vi "浊度电极校准.vi"() -> ()   [LabVIEW 2016, in "斯坦道多参数.lvlib"]
uses:
  <vilib>/Utility/miscctls.llb/LVPointTypeDef.ctl
  <vilib>/Utility/miscctls.llb/LVPositionTypeDef.ctl
  <vilib>/Analysis/NI_AALBase.lvlib
panel:
  in  "刷新按钮":bool
  out "第三点信号值":dbl
  out "第二点信号值":dbl
  out "第一点信号值":dbl
  out "温度":dbl format="%#.2f"
  out "通讯状态":string
  out "电极状态标志":u16(ring) items=["OK"=0, "第一点校正通过"=1, "第二点校正通过"=2, "悬浮物两点校准第一点校正通过"=11, "悬浮物两点校准第二点校正通过"=12, "浊度三点校正第一点校正通过"=31, "浊度三点校正第二点校正通过"=32, "浊度三点校正第三点校正通过"=33]
  out "第三点校准值":dbl
  out "标液3":dbl
  out "第二点校准值":dbl
  out "第一点校准值":dbl
  in  "校准停止":bool
  in  "校准启动":bool
  in  "校准模式":u16(ring) items=["两点校准", "单点校准", "三点校准"]
  out "最小值":sgl format="%#.2f"
  out "最大值":sgl format="%#.2f"
  out "波形图表":dbl(graph) caption="历史曲线"
  out "mean":dbl caption="均值" format="%#.2f"
  out "standard deviation":dbl caption="标准差" format="%#.2f"
  out "变异系数":dbl format="%#.6f"
  out "测量值":dbl format="%#.2f"
  out "提示":string
  out "标液2":dbl
  out "标液1":dbl
  out "信号值":dbl format="%#.2f"
  out "偏移值补偿":dbl caption="浊度偏移修正值" format="%#.2f"
  out "电极斜率":dbl format="%#.6f"
  out "电极零点":dbl format="%#.6f"
  # "浊度电极设定"
  # "℃"
  # "NTU"
  # "%"
  # "请选择校准模式:"
  # "NTU"
  # "NTU"
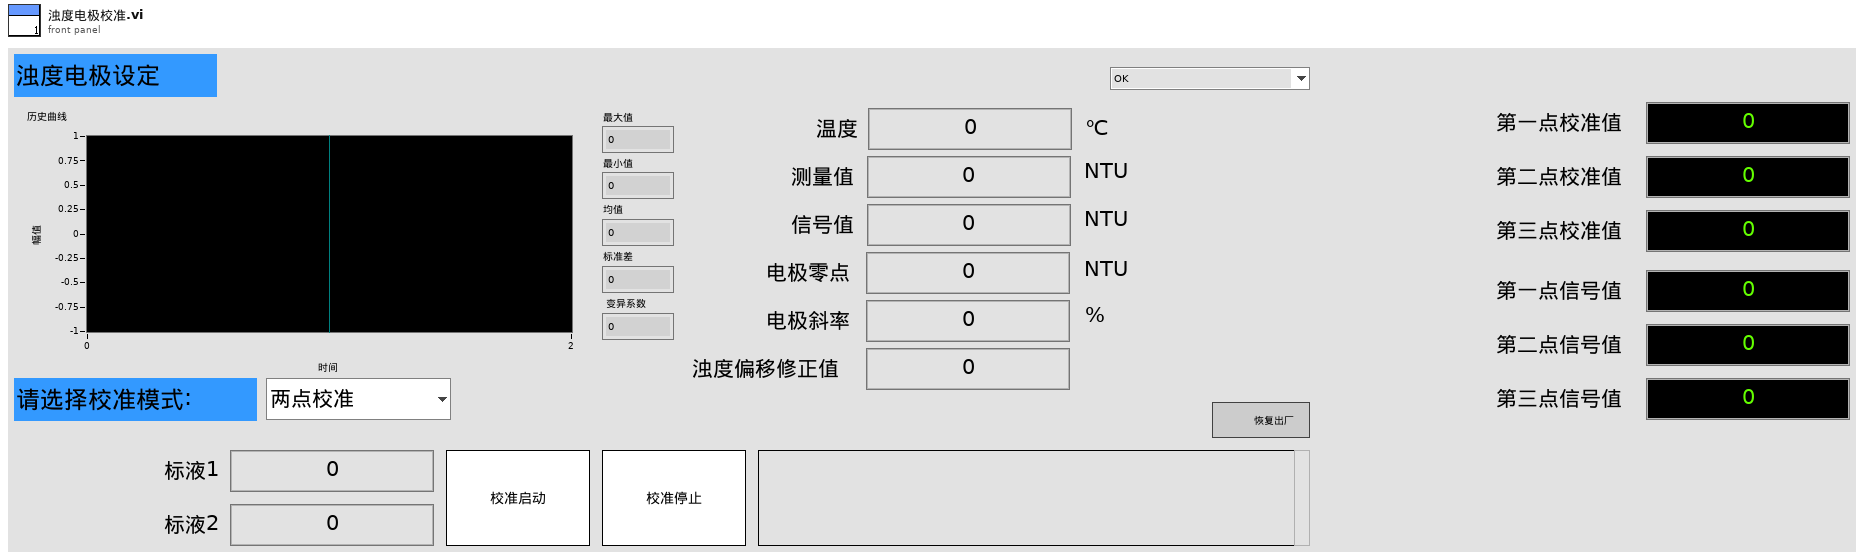
[diagram p1: front panel]
types:
  T1 = typedef "LVPointTypeDef.ctl" = cluster{"Horizontal":i16, "Vertical":i16}
  T2 = cluster{"电极状态标志":u16, "电极型号标志":u16, "浊度测量值":sgl, "温度测量值":sgl, "浊度信号值":sgl, "浊度偏移修正值":sgl, "温度偏移修正值":sgl, "手动温度补偿值":sgl, "浊度电极零点":sgl, "浊度电极斜率":sgl, "第1点标准值记录":sgl, "第1点信号值记录":sgl, "第1点温度值记录":sgl, "第2点标准值记录":sgl, "第2点信号值记录":sgl, "第2点温度值记录":sgl, "命令滤波设定":u16, "温度模式":enum16{"ATC", "MTC"}, "生产批次":u16, "电极序号":u16, "串口地址":u16, "串口波特率":enum16{"9600", "19200", "115200"}, "串口校验位":enum16{"NONE", "ODD", "EVEN"}, "串口停止位":enum16{"1bit", "2bit"}, "第一点标准值":sgl, "第二点标准值":sgl, "第三点标准值":sgl}
  T3 = typedef "LVPositionTypeDef.ctl" = cluster{"Left":i32, "Top":i32}
  T4 = enum8{"Enabled", "Disabled", "Disabled and Grayed Out"}
  T5 = cluster{"测量量程":dbl, "测量精度":dbl, "测量间隔":dbl, "消解温度":dbl, "消解时长":dbl, "空白校准时间":timestamp, "曲线截距":dbl, "曲线斜率":dbl, "测量检出限":dbl, "测量信号值":dbl, "线性相关系数":dbl, "二次多项式系数":dbl, "标样校准时间":timestamp, "单位":enum16{"ug/L", "mg/L"}}
  T6 = cluster{"ph":bool, "DO":bool, "Cond":bool, "Turb":bool, "叶绿素a":bool, "藻密度":bool, "ORP":bool}
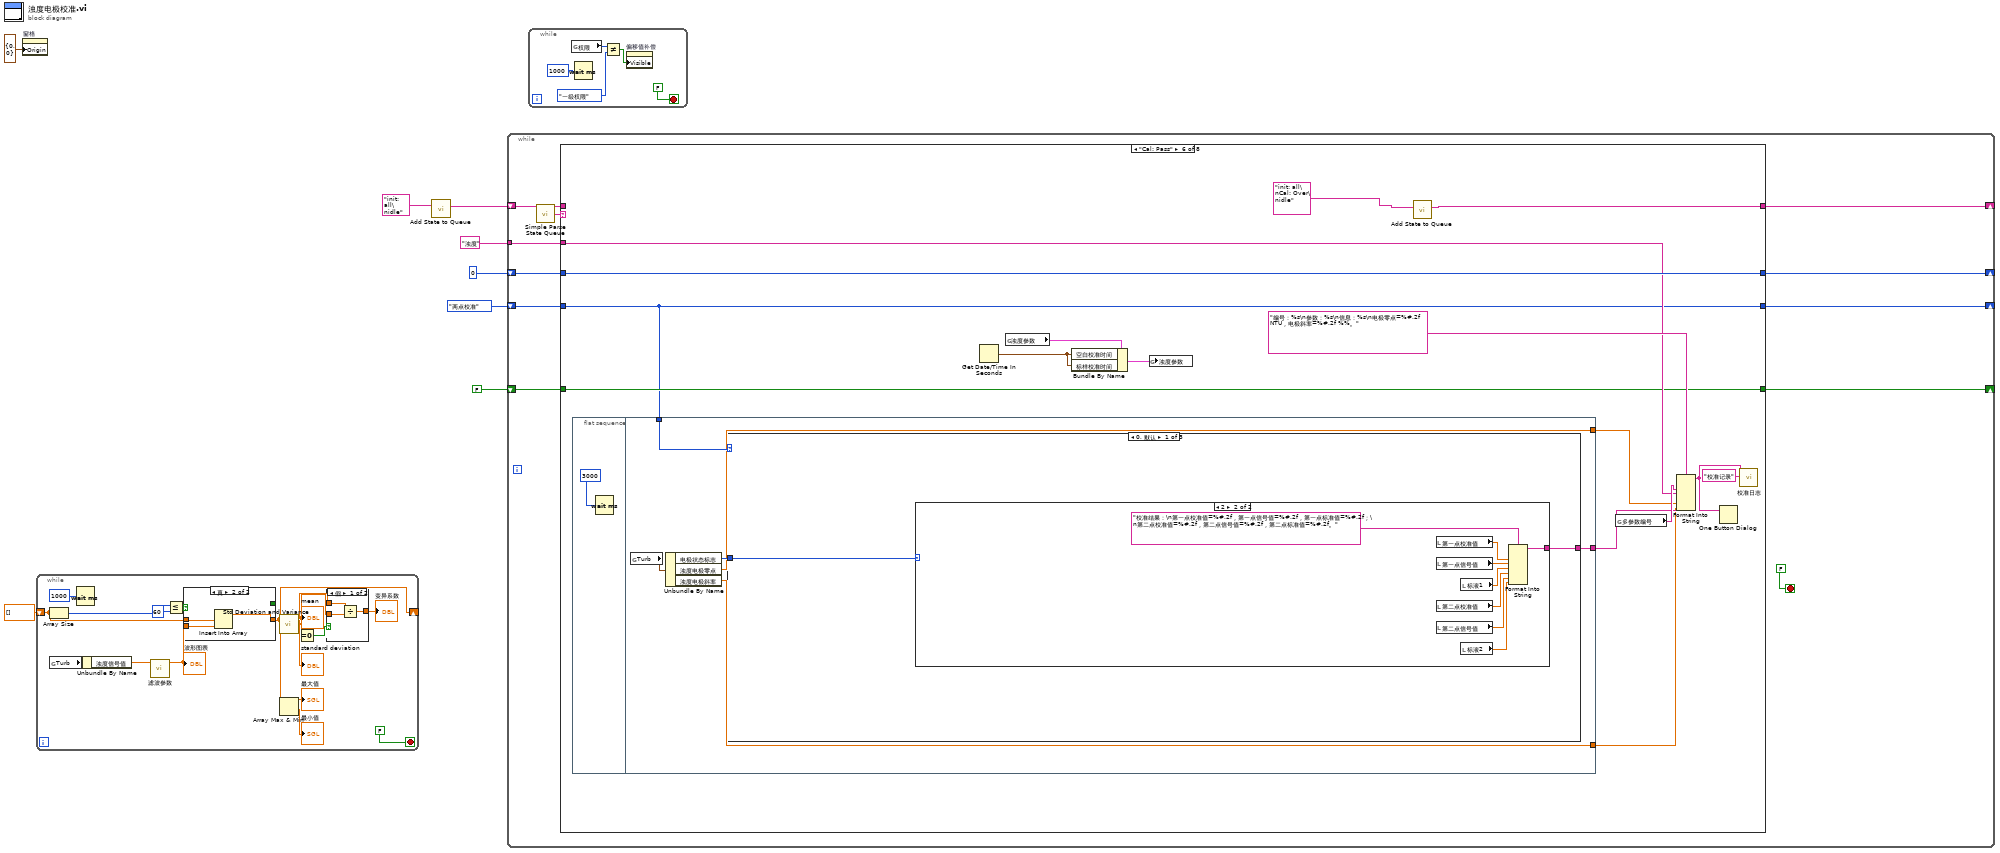
[diagram p0: block diagram]
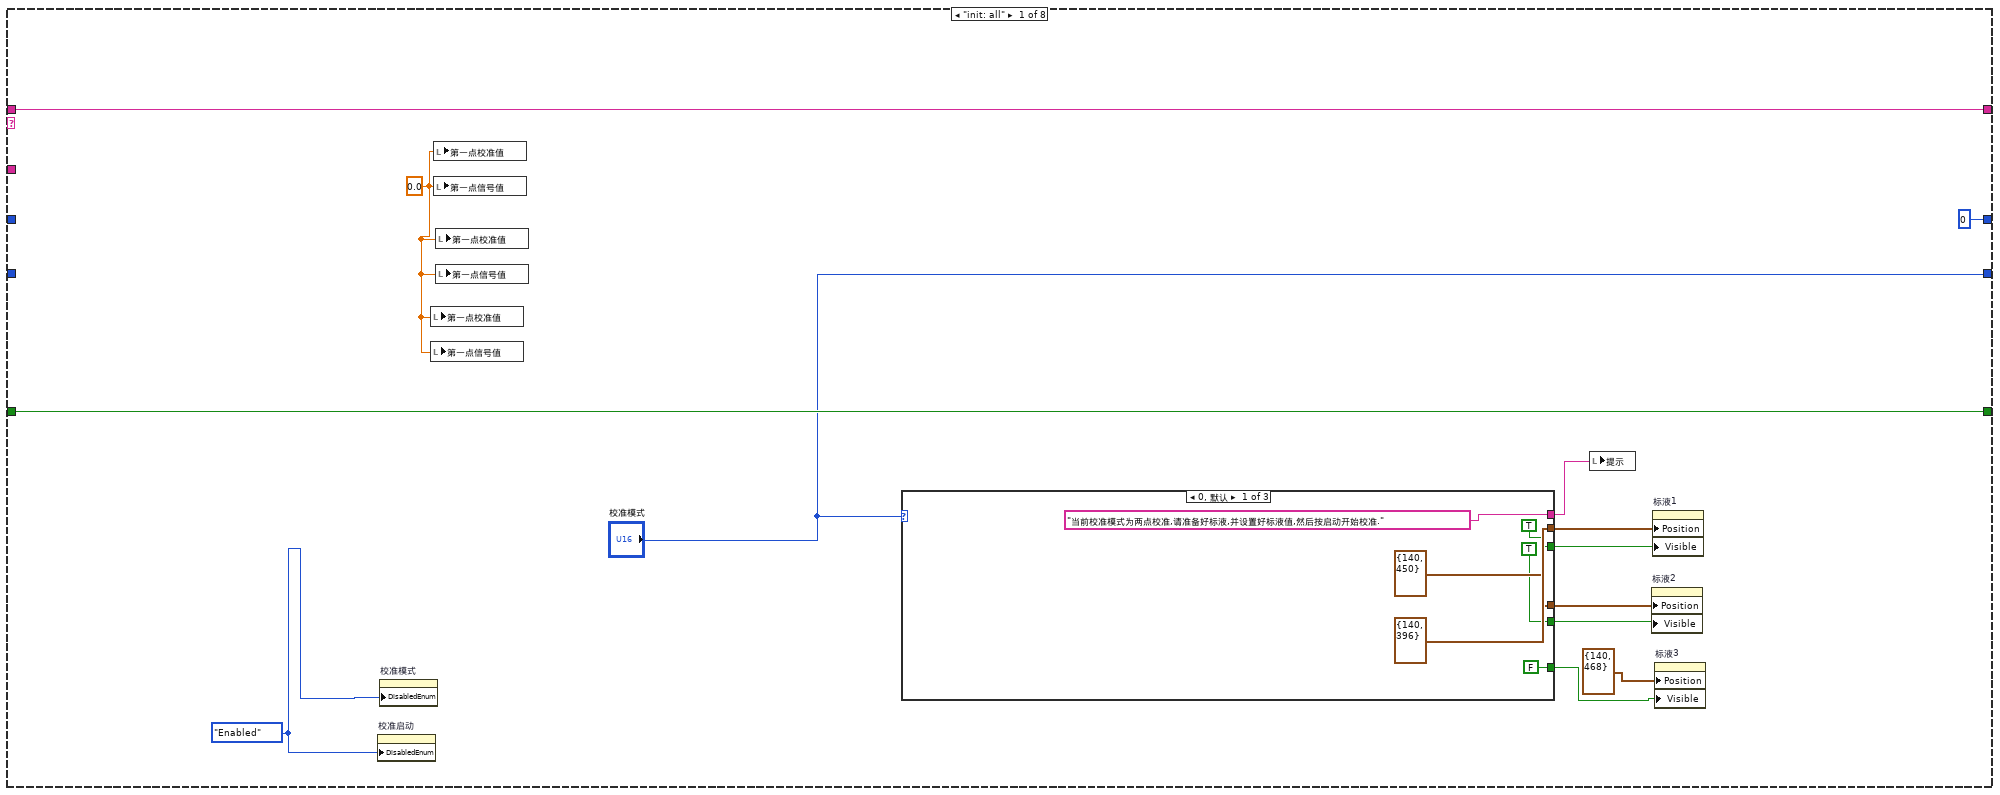
[diagram p2: hidden frame]
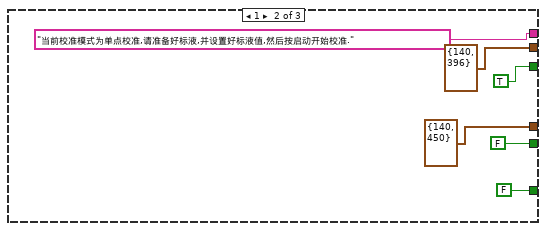
[diagram p3: hidden frame]
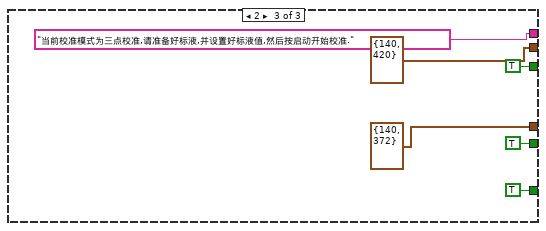
[diagram p4: hidden frame]
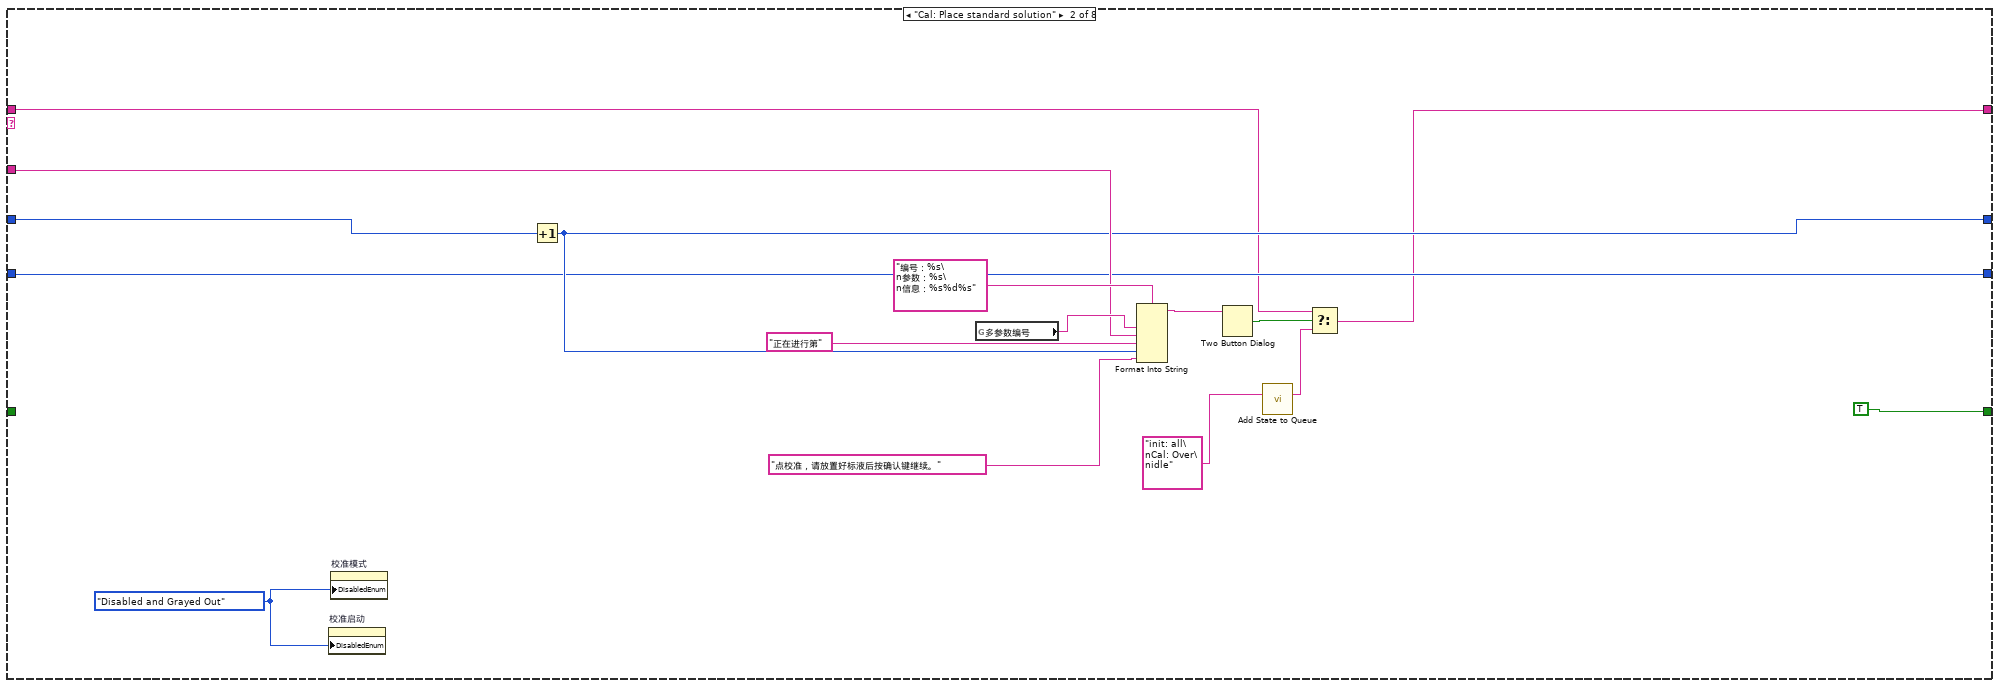
[diagram p5: hidden frame]
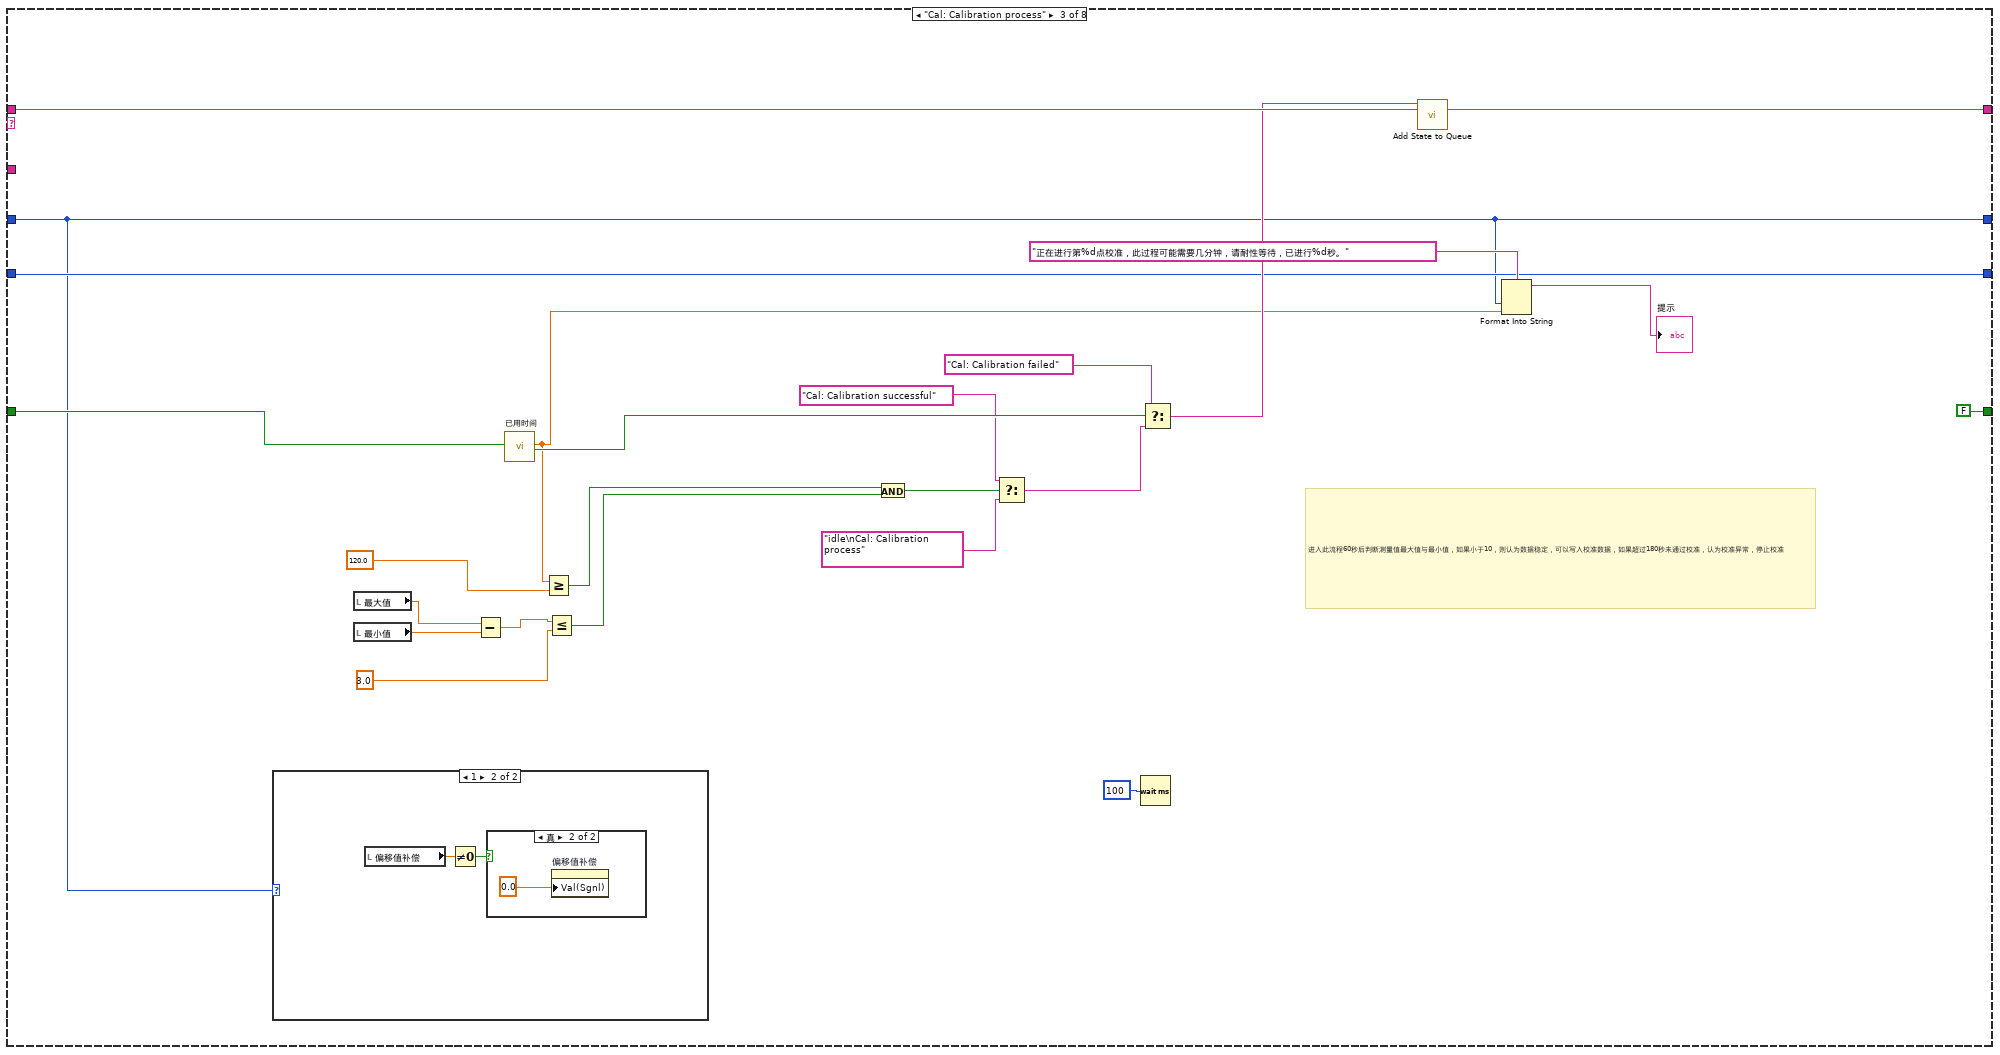
[diagram p6: hidden frame]
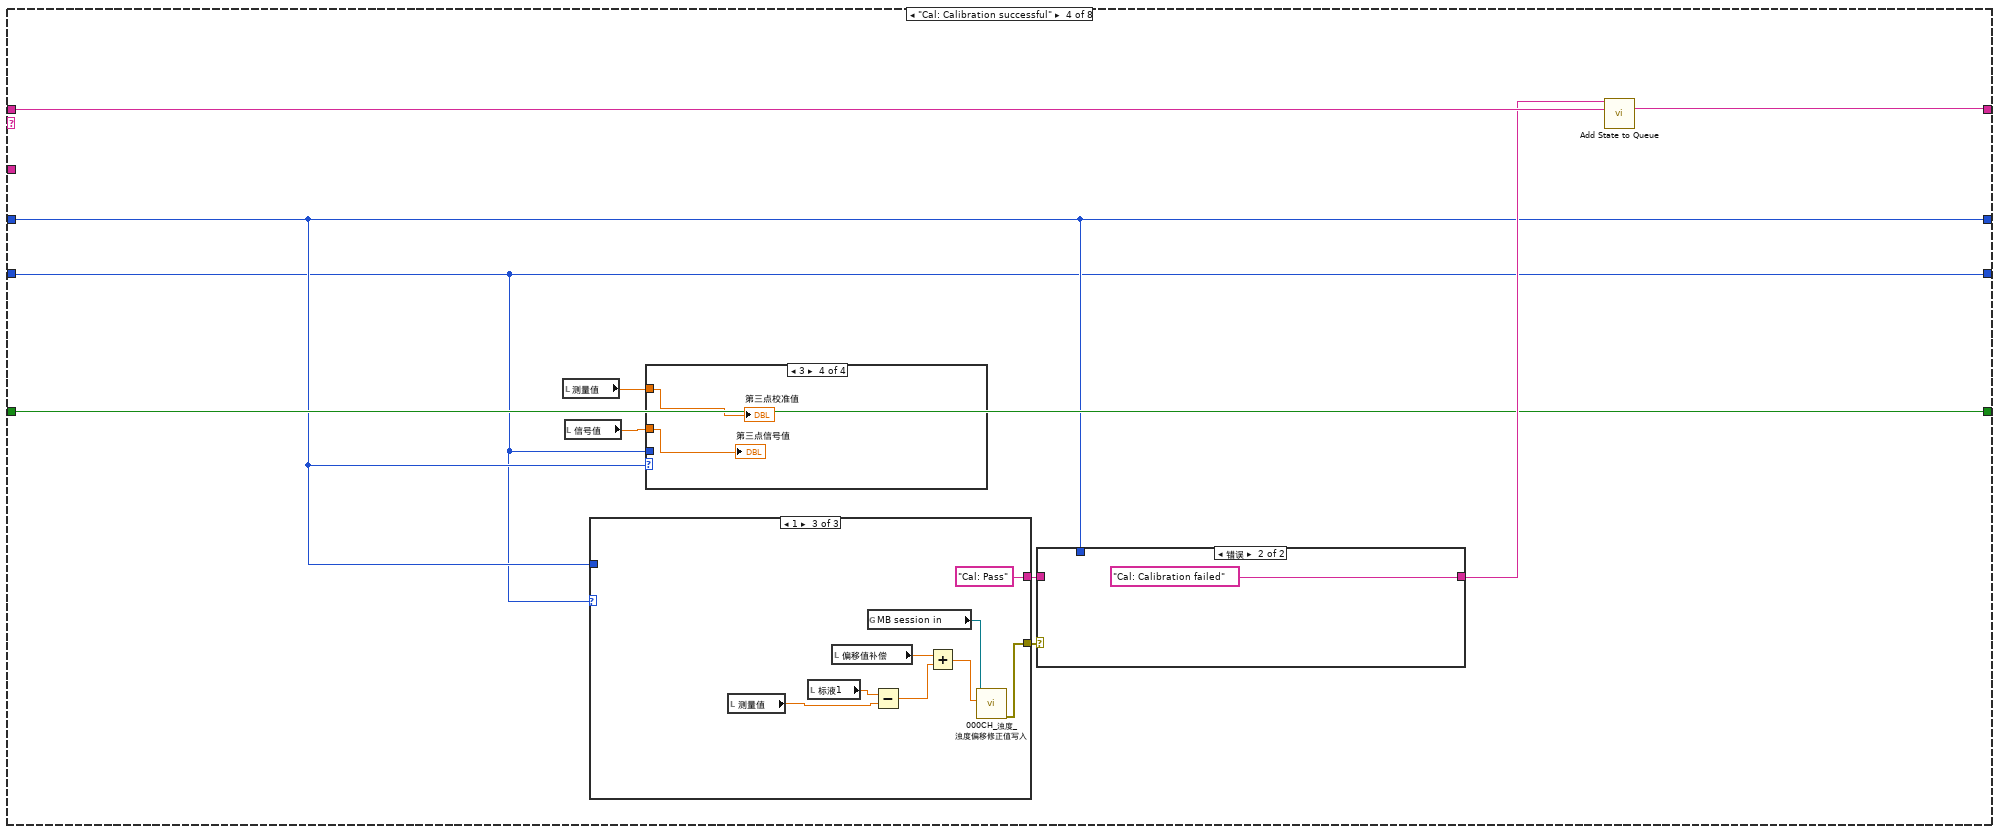
[diagram p9: hidden frame]
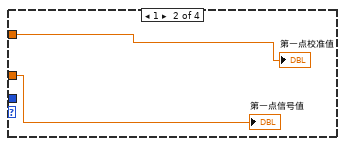
[diagram p11: hidden frame]
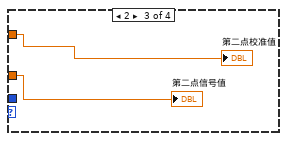
[diagram p12: hidden frame]
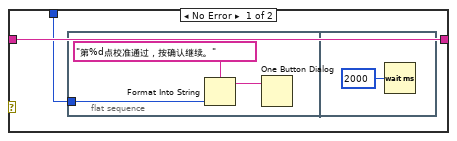
[diagram p13: hidden frame]
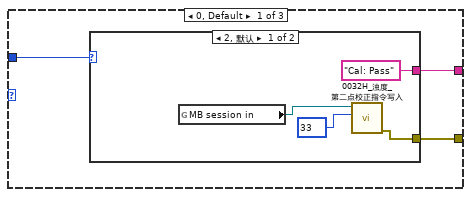
[diagram p14: hidden frame]
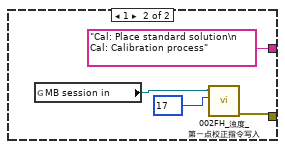
[diagram p15: hidden frame]
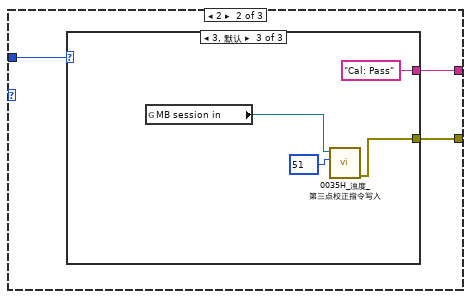
[diagram p16: hidden frame]
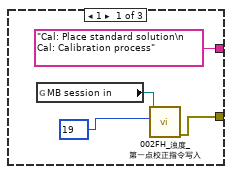
[diagram p17: hidden frame]
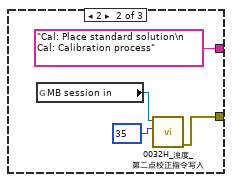
[diagram p18: hidden frame]
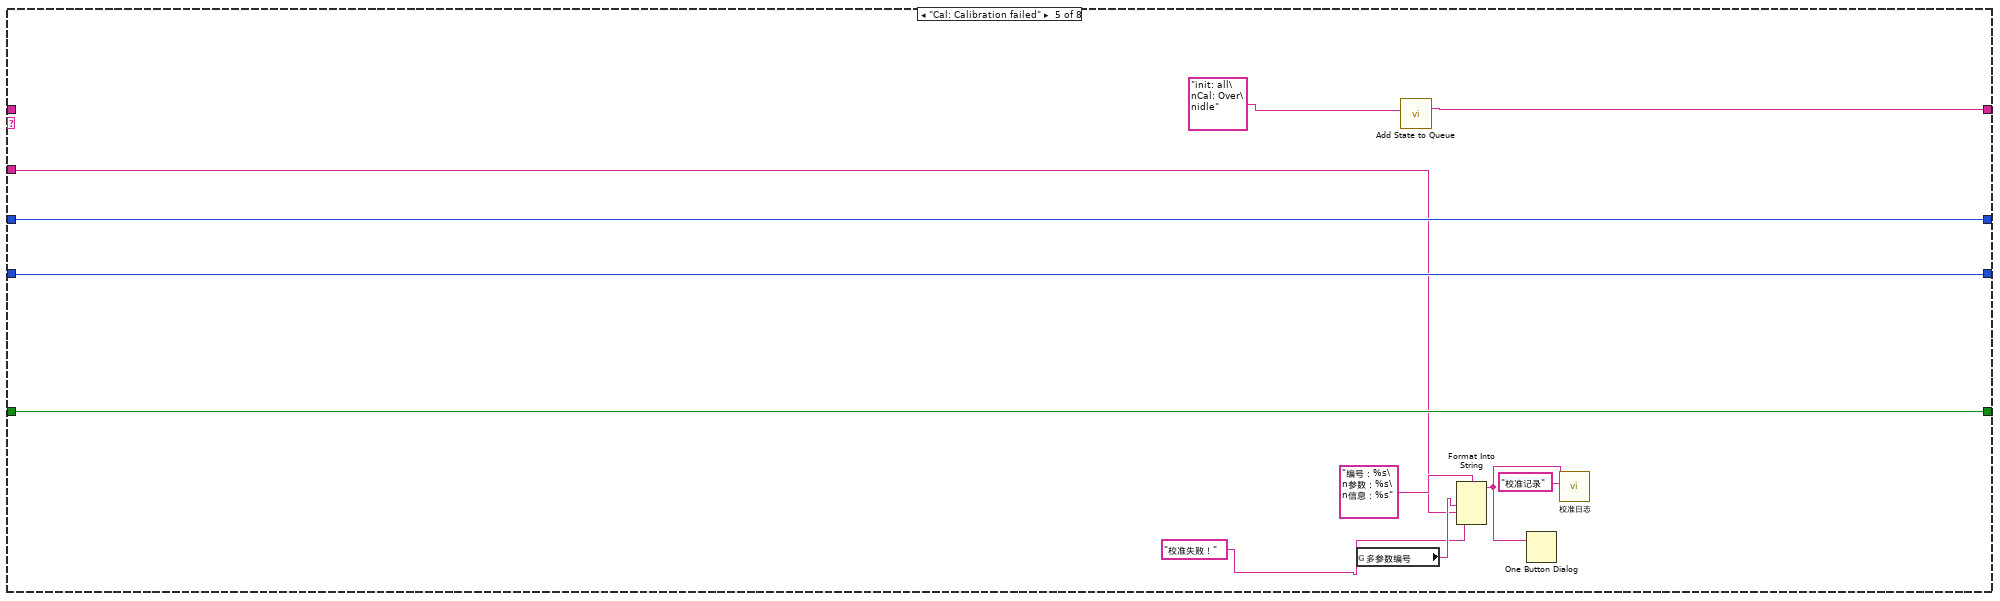
[diagram p19: hidden frame]
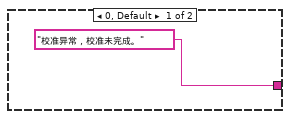
[diagram p20: hidden frame]
diagram:
  n1 = property on="窗格" class="Pane"("Origin"=T1 {"Horizontal"=0, "Vertical"=0} ("原点")) -> ()  [unwired: 2 in, 2 out]
  n2 = while {
    shift-right: [w13] -> _
    shift-left: sgl[] [] -> [w20]
    stop <- FALSE stop-if-true
    n3 = Array Size(array=w20) -> (size(s)=w22:i32)
    n4 = global read "国弘过程全局变量.vi" "Turb"() -> (w14:T2)
    n5 = Wait (ms)(milliseconds to wait=u32 1000 ("等待时间（毫秒）")) -> ()  [unwired: 1 out]
    n6 = Unbundle By Name(w14) -> ("浊度信号值"=w10:sgl)
    n7 = call "滤波参数.vi"("x"=w10) -> ("mode"=w9:dbl)  [unwired: 10 in]
    "波形图表" <- w9
    n8 = Less Or Equal?(x=w22, y=60) -> (x <= y?=w21:bool)
    n9 = case shown="真" w21 {
      tunnel: w20 -> [w33 w36]
      tunnel: w9 -> [w31 w35]
      tunnel: [w29 w34] -> w13
      tunnel: [TRUE _] -> _
      frame False {
        n10 = Replace Array Subset(array=w33, new element=w31) -> (w32:sgl[])  [unwired: 1 in]
        n11 = Rotate 1D Array(1:w32, 2:-1 ("n")) -> (0:w29:sgl[])
      }
      frame True {
        n12 = Insert Into Array(array=w36, new element=w35) -> (w34:sgl[])  [unwired: 1 in]
      }
    }
    n13 = call <vilib>:"Std Deviation and Variance.vi"("X"=w13) -> ("mean"=w18:dbl, "standard deviation"=w17:dbl)  [unwired: 1 in, 1 out]
    "mean" <- w18
    "standard deviation" <- w17
    n14 = Array Max & Min(array=w13) -> (max value=→"最大值":sgl, min value=→"最小值":sgl)  [unwired: 2 out]
    n15 = Equal To 0?(x=w18) -> (x = 0?=w19:bool)
    n16 = case shown="假" w19 {
      tunnel: w17 -> [w27 _]
      tunnel: [w26 _] -> w16
      tunnel: w18 -> [w25 _]
      frame False {
        n17 = Divide(x=w27, y=w25) -> (x/y=w26:dbl)
      }
      frame True {
      }
    }
    "变异系数" <- w16
  }
  n18 = call "Add State to Queue.vi"("State(s) In (\"\")"="init: all\nidle" ("State(s) In (\"\")")) -> ("States Out"=w5:string)  [unwired: 14 in]
  n19 = while {
    shift-right: [w44] -> _
    shift-left: w5 -> [w48]
    shift-right: [w41] -> _
    shift-left: 0 -> [w43]
    tunnel: "浊度" ("State(s) In (\"\")") -> [w42]
    shift-right: [w39] -> _
    shift-left: enum16{"两点校准", "单点校准", "三点校准"}."两点校准" ("校准模式") -> [w40]
    shift-right: [w37] -> _
    shift-left: FALSE -> [w38]
    stop <- FALSE stop-if-true
    n20 = call "Simple Parse State Queue.vi"("State Queue"=w48) -> ("Remain States"=w45:string, "Next State"=w46:string)  [unwired: 13 in]
    n21 = case shown="\"Cal: Pass\"" w46 {
      tunnel: w45 -> [w61 w83 w114 w130 _ _ w247 w257]
      tunnel: [w61 w82 w113 w129 w187 w197 w247 w256] -> w44
      tunnel: w43 -> [_ w91 w98 w124 w190 w206 w246 w254]
      tunnel: w42 -> [_ w92 _ _ w181 w202 _ _]
      tunnel: [0 w89 w98 w124 w190 w206 w246 w255] -> w41
      tunnel: w40 -> [_ w88 w99 w123 w189 w198 w245 w253]
      tunnel: ["校准模式" w88 w99 w123 w189 w198 w245 w253] -> w39
      tunnel: w38 -> [w58 _ w101 w125 w188 w201 w244 w251]
      tunnel: [w58 TRUE FALSE w125 w188 w201 w244 w251] -> w37
      frame "init: all" {
        w56 = T4."Enabled" ("禁用")
        w57 = 0.0 ("第一点校准值")
        n22 = property on="校准启动" class="Bool"("DisabledEnum"=w56) -> ()  [unwired: 2 in, 2 out]
        n23 = property on="校准模式" class="Ring (严格)"("DisabledEnum"=w56) -> ()  [unwired: 2 in, 2 out]
        n24 = local write "第一点校准值"(w57) -> ()
        n25 = local write "第一点信号值"(w57) -> ()
        n26 = local write "第一点校准值"(w57) -> ()
        n27 = local write "第一点信号值"(w57) -> ()
        n28 = local write "第一点校准值"(w57) -> ()
        n29 = local write "第一点信号值"(w57) -> ()
        n30 = case shown="0, 默认" "校准模式" {
          tunnel: ["当前校准模式为两点校准,请准备好标液,并设置好标液值,然后按启动开始校准." ("提示") "当前校准模式为单点校准,请准备好标液,并设置好标液值,然后按启动开始校准." ("提示") "当前校准模式为三点校准,请准备好标液,并设置好标液值,然后按启动开始校准." ("提示")] -> w60
          tunnel: [T3 {"Left"=140, "Top"=396} ("位置") T3 {"Left"=140, "Top"=396} ("位置") T3 {"Left"=140, "Top"=420} ("位置 2")] -> w54
          tunnel: [TRUE ("可见") TRUE ("可见") TRUE ("可见")] -> w53
          tunnel: [FALSE ("可见") FALSE ("可见") TRUE ("可见")] -> w51
          tunnel: [TRUE ("可见") FALSE ("可见") TRUE ("可见")] -> w50
          tunnel: [T3 {"Left"=140, "Top"=450} ("位置 2") T3 {"Left"=140, "Top"=450} ("位置 2") T3 {"Left"=140, "Top"=372} ("位置")] -> w49
          frame 0, Default {
          }
          frame 1 {
          }
          frame 2 {
          }
        }
        n31 = local write "提示"(w60) -> ()
        n32 = property on="标液2" class="DigNum (严格)"("Position"=w49, "Visible"=w50) -> ()  [unwired: 2 in, 2 out]
        n33 = property on="标液1" class="DigNum (严格)"("Position"=w54, "Visible"=w53) -> ()  [unwired: 2 in, 2 out]
        n34 = property on="标液3" class="DigNum (严格)"("Position"=T3 {"Left"=140, "Top"=468} ("位置 3"), "Visible"=w51) -> ()  [unwired: 2 in, 2 out]
      }
      frame "Cal: Place standard solution" {
        w81 = T4."Disabled and Grayed Out" ("禁用")
        n35 = property on="校准启动" class="Bool"("DisabledEnum"=w81) -> ()  [unwired: 2 in, 2 out]
        n36 = property on="校准模式" class="Ring (严格)"("DisabledEnum"=w81) -> ()  [unwired: 2 in, 2 out]
        n37 = Increment(x=w91) -> (x+1=w89:i32)
        n38 = global read "多参数全局变量.vi" "多参数编号"() -> (w94:string)
        n39 = Format Into String(format string="编号：%s\n参数：%s\n信息：%s%d%s" ("格式字符串"), w94, w92, "正在进行第" ("消息"), w89, "点校准，请放置好标液后按确认键继续。" ("消息")) -> (resulting string=w86:string)  [unwired: 2 in, 1 out]
        n40 = Two Button Dialog(message=w86) -> (T button?=w85:bool)  [unwired: 2 in]
        n41 = call "Add State to Queue.vi"("State(s) In (\"\")"="init: all\nCal: Over\nidle" ("State(s) In (\"\")")) -> ("States Out"=w84:string)  [unwired: 14 in]
        n42 = Select(t=w83, s=w85, f=w84) -> (s? t:f=w82:string)
      }
      frame "Cal: Calibration process" {
        # "进入此流程60秒后判断测量值最大值与最小值，如果小于10，则认为数据稳定，可以写入校准数据，如果超过180秒未通过校准，认为校准异常，停止校准"
        n43 = case shown="1" w98 {
          frame 0, Default {
          }
          frame 1 {
            n44 = local read "偏移值补偿"() -> (w120:dbl)
            n45 = Not Equal To 0?(x=w120) -> (x != 0?=w121:bool)
            n46 = case shown="真" w121 {
              frame False {
              }
              frame True {
                n47 = property on="偏移值补偿" class="DigNum (严格)"("Val(Sgnl)"=0.0 ("值(信号)")) -> ()  [unwired: 2 in, 2 out]
              }
            }
          }
        }
        n48 = local read "最大值"() -> (w118:sgl)
        n49 = local read "最小值"() -> (w117:sgl)
        n50 = Subtract(x=w118, y=w117) -> (x-y=w119:sgl)
        n51 = call "已用时间"("Reset"=w101) -> ("Elapsed Time (s)"=w97:dbl, "Time has Elapsed"=w115:bool)  [unwired: 11 in, 6 out]
        n52 = Greater Or Equal?(x=w97, y=120.0) -> (x >= y?=w110:bool)
        n53 = Less Or Equal?(x=w119, y=3.0) -> (x <= y?=w106:bool)
        n54 = And(x=w110, y=w106) -> (x .and. y?=w107:bool)
        n55 = Select(t="Cal: Calibration successful" ("State(s) In (\"\")"), s=w107, f="idle\nCal: Calibration process" ("State(s) In (\"\")")) -> (s? t:f=w105:string)
        n56 = Wait (ms)(milliseconds to wait=u32 100 ("等待时间（毫秒）")) -> ()  [unwired: 1 out]
        n57 = Select(t="Cal: Calibration failed" ("State(s) In (\"\")"), s=w115, f=w105) -> (s? t:f=w104:string)
        n58 = call "Add State to Queue.vi"("State(s) In Front (\"\")"=w104, "State(s) In (\"\")"=w114) -> ("States Out"=w113:string)  [unwired: 13 in]
        n59 = Format Into String(format string="正在进行第%d点校准，此过程可能需要几分钟，请耐性等待，已进行%d秒。" ("格式字符串"), w98, w97) -> (resulting string=→"提示":string)  [unwired: 2 in, 1 out]
      }
      frame "Cal: Calibration successful" {
        n60 = local read "测量值"() -> (w126:dbl)
        n61 = local read "信号值"() -> (w127:dbl)
        n62 = case shown="1" w123 {
          tunnel: [w148 w159 w172] -> w132
          tunnel: [w147 w157 "Cal: Pass" ("State(s) In (\"\")")] -> w131
          tunnel: w124 -> [w146 w158 _]
          frame 0, Default {
            n63 = case shown="2, 默认" w146 {
              tunnel: [w151 w155] -> w148
              tunnel: ["Cal: Pass" ("State(s) In (\"\")") "Cal: Place standard solution\n Cal: Calibration process" ("State(s) In (\"\")")] -> w147
              frame 2, Default {
                n64 = global read "多参数全局变量.vi" "MB session in"() -> (w150:refnum<class "MB_Master.lvclass">)
                n65 = call "0032H_浊度_第二点校正指令写入.vi"("数值"=u16 33, "MB session in"=w150) -> ("error out"=w151:errorcluster)  [unwired: 8 in, 1 out]
              }
              frame 1 {
                n66 = global read "多参数全局变量.vi" "MB session in"() -> (w154:refnum<class "MB_Master.lvclass">)
                n67 = call "002FH_浊度_第一点校正指令写入.vi"("数值"=u16 17, "MB session in"=w154) -> ("error out"=w155:errorcluster)  [unwired: 8 in, 1 out]
              }
            }
          }
          frame 2 {
            n68 = case shown="3, 默认" w158 {
              tunnel: [w162 w165 w169] -> w159
              tunnel: ["Cal: Place standard solution\n Cal: Calibration process" ("State(s) In (\"\")") "Cal: Place standard solution\n Cal: Calibration process" ("State(s) In (\"\")") "Cal: Pass" ("State(s) In (\"\")")] -> w157
              frame 1 {
                n69 = global read "多参数全局变量.vi" "MB session in"() -> (w161:refnum<class "MB_Master.lvclass">)
                n70 = call "002FH_浊度_第一点校正指令写入.vi"("数值"=u16 19, "MB session in"=w161) -> ("error out"=w162:errorcluster)  [unwired: 8 in, 1 out]
              }
              frame 2 {
                n71 = global read "多参数全局变量.vi" "MB session in"() -> (w164:refnum<class "MB_Master.lvclass">)
                n72 = call "0032H_浊度_第二点校正指令写入.vi"("数值"=u16 35, "MB session in"=w164) -> ("error out"=w165:errorcluster)  [unwired: 8 in, 1 out]
              }
              frame 3, Default {
                n73 = global read "多参数全局变量.vi" "MB session in"() -> (w168:refnum<class "MB_Master.lvclass">)
                n74 = call "0035H_浊度_第三点校正指令写入.vi"("数值"=u16 51, "MB session in"=w168) -> ("error out"=w169:errorcluster)  [unwired: 8 in, 1 out]
              }
            }
          }
          frame 1 {
            n75 = local read "测量值"() -> (w175:dbl)
            n76 = local read "标液1"() -> (w179:dbl)
            n77 = local read "偏移值补偿"() -> (w177:dbl)
            n78 = global read "多参数全局变量.vi" "MB session in"() -> (w174:refnum<class "MB_Master.lvclass">)
            n79 = Subtract(x=w179, y=w175) -> (x-y=w178:dbl)
            n80 = Add(x=w177, y=w178) -> (x+y=w173:dbl)
            n81 = call "000CH_浊度_浊度偏移修正值写入.vi"("数值"=w173, "MB session in"=w174) -> ("error out"=w172:errorcluster)  [unwired: 8 in, 1 out]
          }
        }
        n82 = case shown="3" w124 {
          tunnel: w127 -> [_ w134 w136 w138]
          tunnel: w126 -> [_ w133 w135 w137]
          tunnel: w123 -> [_ _ _ _]
          frame 0, Default {
          }
          frame 1 {
            "第一点信号值" <- w134
            "第一点校准值" <- w133
          }
          frame 2 {
            "第二点信号值" <- w136
            "第二点校准值" <- w135
          }
          frame 3 {
            "第三点信号值" <- w138
            "第三点校准值" <- w137
          }
        }
        n83 = case shown="错误" w132 {
          tunnel: w131 -> [w140 _]
          tunnel: [w140 "Cal: Calibration failed" ("State(s) In (\"\")")] -> w128
          tunnel: w124 -> [w139 _]
          frame No Error {
            n84 = flat-sequence {
              tunnel: w139 -> [w141]
              frame #0 {
                n85 = Format Into String(format string="第%d点校准通过，按确认继续。" ("格式字符串"), w141) -> (resulting string=w143:string)  [unwired: 2 in, 1 out]
                n86 = One Button Dialog(message=w143) -> ()  [unwired: 1 in, 1 out]
              }
              frame #1 {
                n87 = Wait (ms)(milliseconds to wait=u32 2000 ("等待时间（毫秒）")) -> ()  [unwired: 1 out]
              }
            }
          }
          frame Error {
          }
        }
        n88 = call "Add State to Queue.vi"("State(s) In Front (\"\")"=w128, "State(s) In (\"\")"=w130) -> ("States Out"=w129:string)  [unwired: 13 in]
      }
      frame "Cal: Calibration failed" {
        n89 = global read "多参数全局变量.vi" "多参数编号"() -> (w184:string)
        n90 = call "Add State to Queue.vi"("State(s) In (\"\")"="init: all\nCal: Over\nidle" ("State(s) In (\"\")")) -> ("States Out"=w187:string)  [unwired: 14 in]
        n91 = Format Into String(format string="编号：%s\n参数：%s\n信息：%s" ("格式字符串"), w184, w181, "校准失败！" ("消息")) -> (resulting string=w183:string)  [unwired: 2 in, 1 out]
        n92 = One Button Dialog(message=w183) -> ()  [unwired: 1 in, 1 out]
        n93 = call "校准日志.vi"("table"="校准记录", "日志信息"=w183) -> ()  [unwired: 9 in, 1 out]
      }
      frame "Cal: Pass" {
        n94 = flat-sequence {
          tunnel: [w211] -> w199
          tunnel: w198 -> [w210]
          tunnel: [w209] -> w196
          tunnel: [w208] -> w195
          frame #0 {
            n95 = Wait (ms)(milliseconds to wait=u32 3000 ("等待时间（毫秒）")) -> ()  [unwired: 1 out]
          }
          frame #1 {
            n96 = global read "国弘过程全局变量.vi" "Turb"() -> (w212:T2)
            n97 = Unbundle By Name(w212) -> ("电极状态标志"=w213:u16, "浊度电极零点"=w209:sgl, "浊度电极斜率"=w208:sgl)
            n98 = case shown="0, 默认" w210 {
              tunnel: [w215 w226 w243] -> w211
              tunnel: w213 -> [w214 w225 _]
              frame 0, Default {
                n99 = case shown="2" w214 {
                  tunnel: ["校准异常，校准未完成。" ("格式字符串") w224] -> w215
                  frame 0, Default {
                  }
                  frame 2 {
                    n100 = local read "第一点校准值"() -> (w222:dbl)
                    n101 = local read "第一点信号值"() -> (w223:dbl)
                    n102 = local read "第二点校准值"() -> (w219:dbl)
                    n103 = local read "第二点信号值"() -> (w218:dbl)
                    n104 = local read "标液1"() -> (w220:dbl)
                    n105 = local read "标液2"() -> (w217:dbl)
                    n106 = Format Into String(format string="校准结果：\n第一点校准值=%#.2f，第一点信号值=%#.2f，第一点标准值=%#.2f；\n第二点校准值=%#.2f，第二点信号值=%#.2f，第二点标准值=%#.2f。" ("提示"), w222, w223, w220, w219, w218, w217) -> (resulting string=w224:string)  [unwired: 2 in, 1 out]
                  }
                }
              }
              frame 2 {
                n107 = case shown="33" w225 {
                  tunnel: ["校准异常，校准未完成。" ("格式字符串") w238] -> w226
                  frame 0, Default {
                  }
                  frame 33 {
                    n108 = local read "标液2"() -> (w229:dbl)
                    n109 = local read "标液1"() -> (w230:dbl)
                    n110 = local read "第一点校准值"() -> (w237:dbl)
                    n111 = local read "第一点信号值"() -> (w235:dbl)
                    n112 = local read "第二点校准值"() -> (w234:dbl)
                    n113 = local read "第二点信号值"() -> (w233:dbl)
                    n114 = local read "第三点校准值"() -> (w232:dbl)
                    n115 = local read "第三点信号值"() -> (w231:dbl)
                    n116 = local read "标液3"() -> (w228:dbl)
                    n117 = Format Into String(format string="校准结果：\n第一点校准值=%#.2f，第一点信号值=%#.2f，第一点标准值=%#.2f；\n第二点校准值=%#.2f，第二点信号值=%#.2f，第二点标准值=%#.2f；\n第三点校准值=%#.2f，第三点信号值=%#.2f，第三点标准值=%#.2f。" ("提示"), w237, w235, w230, w234, w233, w229, w232, w231, w228) -> (resulting string=w238:string)  [unwired: 2 in, 1 out]
                  }
                }
              }
              frame 1 {
                n118 = local read "第一点校准值"() -> (w242:dbl)
                n119 = local read "第一点信号值"() -> (w240:dbl)
                n120 = local read "标液1"() -> (w239:dbl)
                n121 = Format Into String(format string="校准结果：\n校准值=%#.2f，信号值=%#.2f，标准值=%#.2f。" ("提示"), w242, w240, w239) -> (resulting string=w243:string)  [unwired: 2 in, 1 out]
              }
            }
          }
        }
        n122 = Get Date/Time In Seconds() -> (seconds since 1Jan1904=w191:timestamp)
        n123 = global read "断电保存变量.vi" "浊度参数"() -> (w193:T5)
        n124 = Bundle By Name(cluster=w193, "空白校准时间"=w191, "标样校准时间"=w191) -> (w192:T5)
        n125 = global write "断电保存变量.vi" "浊度参数"(w192) -> ()
        n126 = call "Add State to Queue.vi"("State(s) In (\"\")"="init: all\nCal: Over\nidle" ("State(s) In (\"\")")) -> ("States Out"=w197:string)  [unwired: 14 in]
        n127 = global read "多参数全局变量.vi" "多参数编号"() -> (w203:string)
        n128 = Format Into String(format string="编号：%s\n参数：%s\n信息：%s\n电极零点=%#.2f NTU，电极斜率=%#.2f %%。" ("格式字符串"), w203, w202, w199, w196, w195) -> (resulting string=w200:string)  [unwired: 2 in, 1 out]
        n129 = One Button Dialog(message=w200) -> ()  [unwired: 1 in, 1 out]
        n130 = call "校准日志.vi"("table"="校准记录", "日志信息"=w200) -> ()  [unwired: 9 in, 1 out]
      }
      frame "Cal: Over" {
        n131 = global read "多参数全局变量.vi" "校准运行状态"() -> (w249:T6)
        n132 = Bundle By Name(cluster=w249, "Turb"=FALSE) -> (w250:T6)
        n133 = global write "多参数全局变量.vi" "校准运行状态"(w250) -> ()
      }
      frame "idle", Default {
        n134 = event shown="[8] \"校准启动\": 值改变" {
          selector: _ -> [_ _ _ _ _ _ _ _ _ _]
          dyn-events: _ -> [_ _ _ _ _ _ _ _ _ _]
          timeout: 10 -> [_ _ _ _ _ _ _ _ _ _]
          tunnel: [_ _ _ w291 w298 w304 w310 _ _ _] -> _
          tunnel: w257 -> [w275 w279 w282 w294 w295 w301 w307 w317 w326 _]
          tunnel: [w274 w278 w283 w293 w299 w305 w311 w316 w325 w328] -> w256
          tunnel: [w273 w276 w284 w292 w300 w306 w312 w315 w323 w329] -> w255
          tunnel: w254 -> [w273 w276 w284 w292 w300 w306 w312 w315 w323 w329]
          event Timeout {
            n135 = event-data() -> ()  [unwired: 1 in, 3 out]
            n136 = global read "国弘过程全局变量.vi" "Turb"() -> (w258:T2)
            n137 = Unbundle By Name(w258) -> ("电极状态标志"=→"电极状态标志":u16, "浊度电极零点"=→"电极零点":sgl, "浊度电极斜率"=→"电极斜率":sgl, "浊度偏移修正值"=→"偏移值补偿":sgl, "浊度信号值"=→"信号值":sgl, "第一点标准值"=→"标液1":sgl, "第二点标准值"=→"标液2":sgl, "浊度测量值"=→"测量值":sgl, "第三点标准值"=→"标液3":sgl, "温度测量值"=→"温度":sgl)  [unwired: 1 out]
            n138 = global read "多参数全局变量.vi" "浊度通讯状态"() -> (w270:bool)
            n139 = property on="通讯状态" class="Str"("Blinking"=TRUE ("闪烁"), "Text.BG Color"=u32 16711680, "Visible"=w270) -> ()  [unwired: 2 in, 2 out]
            n140 = call "Add State to Queue.vi"("State(s) In (\"\")"=w275) -> ("States Out"=w274:string)  [unwired: 14 in]
            "通讯状态" <- "通讯异常" ("当前串口")
          }
          event "校准模式": Value Change {
            n141 = event-data() -> ()  [unwired: 1 in, 6 out]
            n142 = call "Add State to Queue.vi"("State(s) In (\"\")"=w279, "State(s) At Back (\"\")"="init: all\nidle" ("State(s) In (\"\")")) -> ("States Out"=w278:string)  [unwired: 13 in]
          }
          event "偏移值补偿", "标液1", "标液2", "标液3": Mouse Down {
            n143 = event-data() -> ("CtlRef"=w281:refnum<vi>)  [unwired: 1 in, 7 out]
            n144 = property class="DigNum (严格)"(reference=w281) -> ("DisabledEnum"=w280:T4)  [unwired: 1 in, 2 out]
            n145 = case shown="\"Enabled\"" w280 {
              tunnel: w281 -> [w288 _]
              frame "Enabled" {
                n146 = property class="DigNum (严格)"(reference=w288) -> (reference out=w285:refnum<vi>, "Value"=w286:dbl)  [unwired: 1 in, 1 out]
                n147 = call "数字键盘.vi"("OldNumber"=w286) -> ("NewNumber"=w287:dbl)  [unwired: 1 in]
                n148 = property class="DigNum (严格)"(reference=w285, "Val(Sgnl)"=w287) -> ()  [unwired: 1 in, 2 out]
              }
              frame "Disabled", Default {
              }
            }
            n149 = call "Add State to Queue.vi"("State(s) In (\"\")"=w282) -> ("States Out"=w283:string)  [unwired: 14 in]
          }
          event "偏移值补偿": Value Change {
            n150 = event-data() -> ("NewVal"=w289:dbl)  [unwired: 1 in, 5 out]
            n151 = global read "多参数全局变量.vi" "MB session in"() -> (w290:refnum<class "MB_Master.lvclass">)
            n152 = call "000CH_浊度_浊度偏移修正值写入.vi"("数值"=w289, "MB session in"=w290) -> ("error out"=w291:errorcluster)  [unwired: 8 in, 1 out]
            n153 = call "Add State to Queue.vi"("State(s) In (\"\")"=w294) -> ("States Out"=w293:string)  [unwired: 14 in]
          }
          event "标液1": Value Change {
            n154 = event-data() -> ("NewVal"=w296:dbl)  [unwired: 1 in, 5 out]
            n155 = global read "多参数全局变量.vi" "MB session in"() -> (w297:refnum<class "MB_Master.lvclass">)
            n156 = call "0030H_浊度_第一点标准值写入.vi"("数值"=w296, "MB session in"=w297) -> ("error out"=w298:errorcluster)  [unwired: 8 in, 1 out]
            n157 = call "Add State to Queue.vi"("State(s) In (\"\")"=w295) -> ("States Out"=w299:string)  [unwired: 14 in]
          }
          event "标液2": Value Change {
            n158 = event-data() -> ("NewVal"=w302:dbl)  [unwired: 1 in, 5 out]
            n159 = global read "多参数全局变量.vi" "MB session in"() -> (w303:refnum<class "MB_Master.lvclass">)
            n160 = call "0033H_浊度_第二点标准值写入.vi"("数值"=w302, "MB session in"=w303) -> ("error out"=w304:errorcluster)  [unwired: 8 in, 1 out]
            n161 = call "Add State to Queue.vi"("State(s) In (\"\")"=w301) -> ("States Out"=w305:string)  [unwired: 14 in]
          }
          event "标液3": Value Change {
            n162 = event-data() -> ("NewVal"=w308:dbl)  [unwired: 1 in, 5 out]
            n163 = global read "多参数全局变量.vi" "MB session in"() -> (w309:refnum<class "MB_Master.lvclass">)
            n164 = call "0036H_浊度_第三点标准值写入.vi"("数值"=w308, "MB session in"=w309) -> ("error out"=w310:errorcluster)  [unwired: 8 in, 1 out]
            n165 = call "Add State to Queue.vi"("State(s) In (\"\")"=w307) -> ("States Out"=w311:string)  [unwired: 14 in]
          }
          event "刷新按钮": Value Change {
            n166 = event-data() -> ()  [unwired: 1 in, 6 out]
            n167 = call "Add State to Queue.vi"("State(s) In (\"\")"=w317) -> ("States Out"=w316:string)  [unwired: 14 in]
            n168 = Two Button Dialog(message="请再次确实是否恢复出厂设置！" ("消息")) -> (T button?=w314:bool)  [unwired: 2 in]
            n169 = case shown="真" w314 {
              frame False {
              }
              frame True {
                w318 = u16 33 items=["Factory Reset"=33] ("数值")
                n170 = global read "多参数全局变量.vi" "MB session in"() -> (w319:refnum<class "MB_Master.lvclass">)
                n171 = call "0026H_浊度_命令寄存器写入.vi"("数值"=w318, "MB session in"=w319) -> ()  [unwired: 8 in, 2 out]
              }
            }
          }
          event "校准启动": Value Change {
            n172 = event-data() -> ()  [unwired: 1 in, 6 out]
            n173 = global read "多参数全局变量.vi" "校准运行状态"() -> (w321:T6)
            n174 = Bundle By Name(cluster=w321, "Turb"=TRUE) -> (w322:T6)
            n175 = global write "多参数全局变量.vi" "校准运行状态"(w322) -> ()
            n176 = call "Add State to Queue.vi"("State(s) In (\"\")"=w326, "State(s) At Back (\"\")"="init: all\nCal: Place standard solution\n Cal: Calibration process\nidle" ("State(s) In (\"\")")) -> ("States Out"=w325:string)  [unwired: 13 in]
          }
          event "校准停止": Value Change {
            n177 = event-data() -> ()  [unwired: 1 in, 6 out]
            n178 = call "Add State to Queue.vi"("State(s) In (\"\")"="init: all\nCal: Over\nidle" ("State(s) In (\"\")")) -> ("States Out"=w328:string)  [unwired: 14 in]
          }
        }
      }
    }
  }
  n179 = while {
    stop <- FALSE stop-if-true
    n180 = global read "多参数全局变量.vi" "权限"() -> (w333:enum16{"一级权限", "二级权限", "三级权限"})
    n181 = Wait (ms)(milliseconds to wait=u32 1000 ("等待时间（毫秒）")) -> ()  [unwired: 1 out]
    n182 = Not Equal?(x=w333, y=enum16{"一级权限", "二级权限", "三级权限"}."一级权限") -> (x != y?=w331:bool)
    n183 = property on="偏移值补偿" class="DigNum (严格)"("Visible"=w331) -> ()  [unwired: 2 in, 2 out]
  }
